vi "Pcre2PatternInfoNameTablePointer.vi"(8 "error in":errorcluster, 11 "pCode":u64 format="%.0x") -> (0 "error out":errorcluster, 2 "pNameTable":u64 format="%.0x", 3 "pCode":u64 format="%.0x")   [LabVIEW 2021, in "libpcre2-8.lvlib"]
uses:
  libpcre2-8.lvlib
  Pcre2FnkCallError.vi
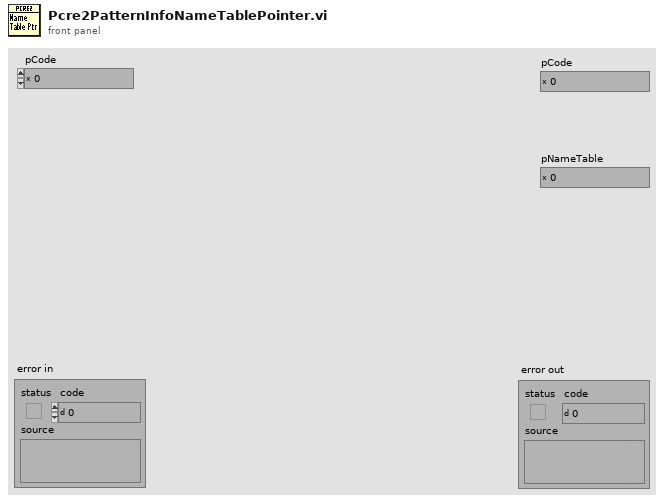
[diagram p1: front panel]
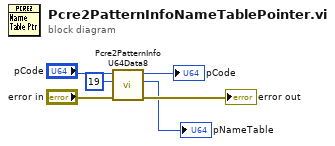
[diagram p0: block diagram]
diagram:
  n1 = call "Pcre2PatternInfoU64Data8.vi"("error in"="error in", "What"=u32 19, "pCode"="pCode") -> ("error out"=→"error out":errorcluster, "Info"=→"pNameTable":u64, "pCode"=→"pCode":u64)  [unwired: 6 in]
